vi "LEDStates.vi"(1 "ButtonInput":bool) -> (0 "Enum":enum16{"Off", "On", "Auto"}(ring)=enum."Auto")   [LabVIEW 2014]
uses:
  <vilib>/ptbypt/NI_PtbyPt.lvlib
panel:
  in  "Stop":bool
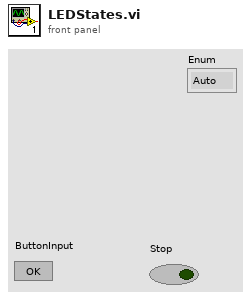
[diagram p1: front panel]
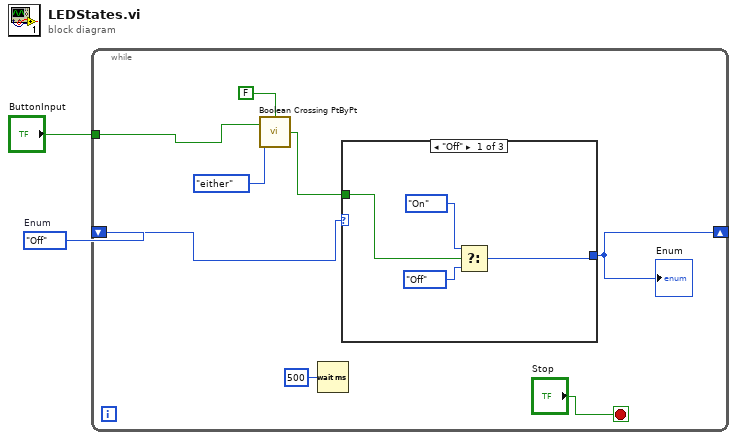
[diagram p0: block diagram]
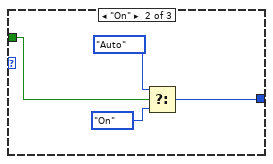
[diagram p2: hidden frame]
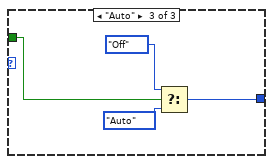
[diagram p3: hidden frame]
diagram:
  w2 = enum16{"Off", "On", "Auto"}."Off"  # Enum
  n1 = while {
    shift-right: [w7] -> _
    shift-left: w2 -> [w8]
    tunnel: "ButtonInput" -> [w3]
    stop <- "Stop" stop-if-true
    n2 = call <vilib>:"Boolean Crossing PtByPt.vi"("initialize"=FALSE, "direction"=enum16{"either", "false-true", "true-false"}."either", "input"=w3) -> ("crossing"=w4:bool)
    n3 = Wait (ms)(milliseconds to wait=u32 500) -> ()  [unwired: 1 out]
    n4 = case shown="\"Off\"" w8 {
      tunnel: [w12 w16 w20] -> w7
      tunnel: w4 -> [w11 w15 w19]
      frame "Off" {
        n5 = Select(t=enum16{"Off", "On", "Auto"}."On", s=w11, f=enum16{"Off", "On", "Auto"}."Off") -> (s? t:f=w12:enum16{"Off", "On", "Auto"})
      }
      frame "On" {
        n6 = Select(t=enum16{"Off", "On", "Auto"}."Auto", s=w15, f=enum16{"Off", "On", "Auto"}."On") -> (s? t:f=w16:enum16{"Off", "On", "Auto"})
      }
      frame "Auto" {
        n7 = Select(t=enum16{"Off", "On", "Auto"}."Off", s=w19, f=enum16{"Off", "On", "Auto"}."Auto") -> (s? t:f=w20:enum16{"Off", "On", "Auto"})
      }
    }
    "Enum" <- w7
  }
